vi "NOR.vi"(1 "b":bool, 2 "a":bool) -> (0 "x":bool)   [LabVIEW 2012]
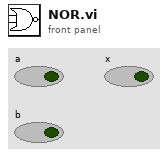
[diagram p1: front panel]
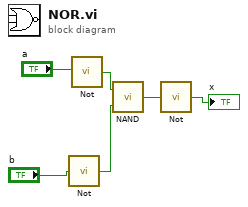
[diagram p0: block diagram]
diagram:
  n1 = call "Not.vi"("In"="b") -> ("Out"=w6:bool)
  n2 = call "Not.vi"("In"="a") -> ("Out"=w5:bool)
  n3 = call "NAND.vi"("b"=w6, "a"=w5) -> ("x"=w2:bool)
  n4 = call "Not.vi"("In"=w2) -> ("Out"=→"x":bool)
